vi "ZPL Config UVP_UVL.vi"(6 "Settle (1 mS)":u32=1, 7 "UVP_UVL selector":bool, 8 "error":errorcluster, 10 "UVL UVP value":dbl format="%.4f", 11 "VISA":refnum<visa-resource-name>) -> (0 "error out":errorcluster, 3 "VISA out":refnum<visa-resource-name>)   [LabVIEW 2015]
doc: "This command sets the under voltage protection (UVP) status of the power supply. If the UVP status is UVP, then the under voltage protection is enabled. If the UVP status is UVL, then the under voltage protection is disabled and only under voltage level (UVL) is enabled\n\nThis VI will wait for \"Settle\" milliseconds after setting the limit to allow the output to reach the new setting. If unwired, there will be no delay"
panel:
  # "Lambda ZPLUS \n Serial Port\n  DC Power Supplies"
  # "Select and Set UVP/UVL"
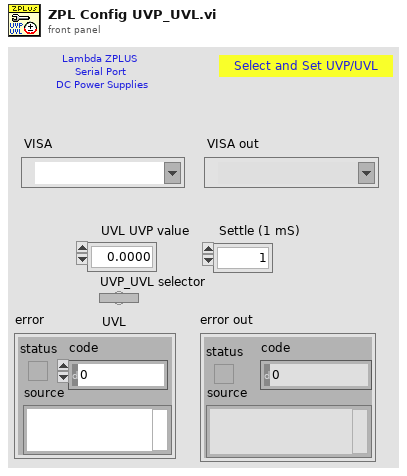
[diagram p1: front panel]
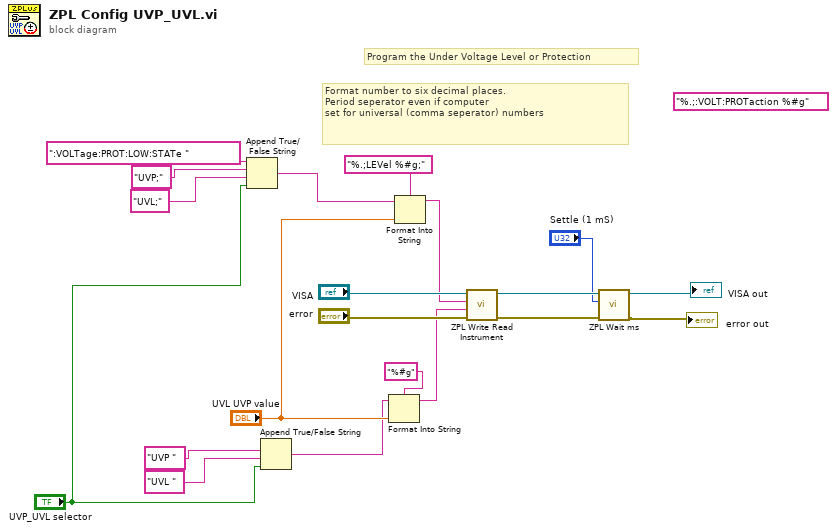
[diagram p0: block diagram]
diagram:
  (unwired) "%.;:VOLT:PROTaction %#g" ("format string")
  # "Format number to six decimal places.\nPeriod seperator even if computer \nset for universal (comma seperator) numbers"
  # "Program the Under Voltage Level or Protection"
  n1 = Append True/False String(1:"UVP_UVL selector", 2:"UVL;" ("true string"), 3:"UVP;" ("true string"), 4:":VOLTage:PROT:LOW:STATe " ("format string")) -> (0:w6:string)
  n2 = Append True/False String(1:"UVP_UVL selector", 2:"UVL " ("true string"), 3:"UVP " ("true string")) -> (0:w3:string)  [unwired: 1 in]
  n3 = Format Into String(format string="%#g", initial string=w3, "UVL UVP value") -> (resulting string=w16:string)  [unwired: 1 in, 1 out]
  n4 = Format Into String(format string="%.;LEVel %#g;", initial string=w6, "UVL UVP value") -> (resulting string=w18:string)  [unwired: 1 in, 1 out]
  n5 = call "ZPL Write Read Instrument.vi"("error in"="error", "Write Command/Query GEN"=w16, "Write Command/Query SCPI"=w18, "VISA"="VISA") -> ("error out"=w13:errorcluster, "VISA  out"=w14:refnum<visa-resource-name>)  [unwired: 5 in, 1 out]
  n6 = call "ZPL Wait ms.vi"("error"=w13, "Delay (1 mS)"="Settle (1 mS)", "VISA"=w14) -> ("error out"=→"error out":errorcluster, "VISA out"=→"VISA out":refnum<visa-resource-name>)  [unwired: 7 in]
